vi "Get CD Item Property Value.vi"(8 "error in (no error)":errorcluster, 10 "CD Item Ref in":T1 format="%.0x", 11 "Double Parameter in":refnum<class "Double Array Parameter.lvclass">) -> (0 "error out":errorcluster, 3 "Double Parameter out":refnum<class "Double Array Parameter.lvclass">)   [LabVIEW 2019, in "CD Parameter Manager API.lvlib" / "Double Array Parameter.lvclass"]
uses:
  Double Array Parameter.lvclass
  C:/Repositories/UI-Control-Initializer-API/Source/Parameter Class/Parameter.lvclass
  <vilib>/NI VeriStand/Custom Device API/Custom Device Item Ref.ctl
  Parameter Class/Parameter.lvclass/Parameter.ctl
  Double Array Parameter.lvclass/Double Array Parameter.ctl
  Parameter Class/Member Accessors/Read Control label.vi
  Member Accessors/Read Value.vi
  Member Accessors/Write Value.vi
  <vilib>/NI VeriStand/Custom Device API/Get Item Property (Double Array).vi
  <vilib>/NI VeriStand/Custom Device API/Custom Device API.lvlib
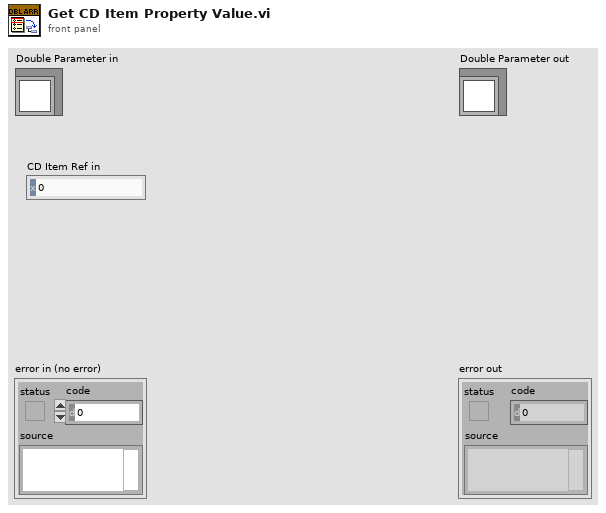
[diagram p1: front panel]
types:
  T1 = typedef "Custom Device API.lvlib/Custom Device Item Ref.ctl" = u64
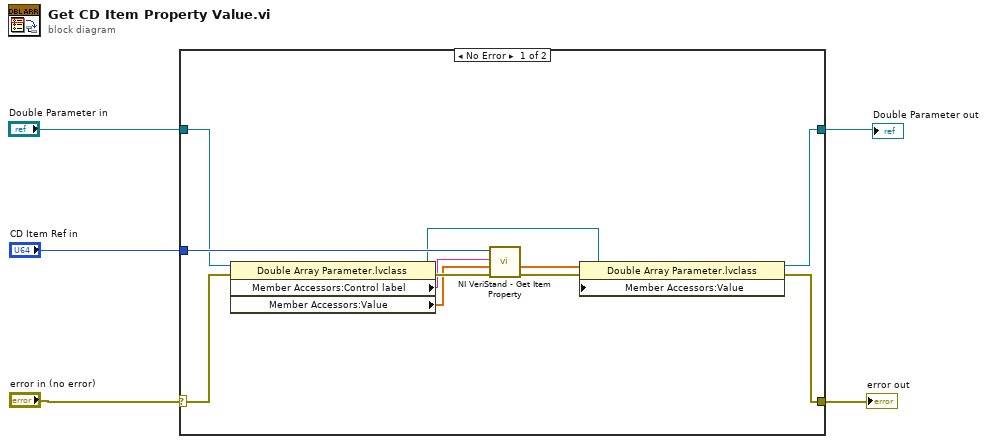
[diagram p0: block diagram]
diagram:
  n1 = case shown="No Error" "error in (no error)" {
    selector: "error in (no error)" -> [w15 w17]
    tunnel: [w11 w17] -> w4
    tunnel: "CD Item Ref in" -> [w16 _]
    tunnel: [w8 w18] -> w5
    tunnel: "Double Parameter in" -> [w7 w18]
    frame No Error {
      n2 = property class="Double Array Parameter.lvclass"(reference=w7, error in=w15) -> (reference out=w9:refnum<class "Double Array Parameter.lvclass">, error out=w14:errorcluster, "Member Accessors:Control label"=w13:string, "Member Accessors:Value"=w6:dbl[])
      n3 = call-poly <vilib>:"NI VeriStand - Get Item Property.vi"("error in (no error)"=w14, "Default Value"=w6, "Property Name"=w13, "Item Ref in"=w16) -> ("error out"=w12:errorcluster, "Value"=w10:dbl[])  [unwired: 4 in, 2 out]
      n4 = property class="Double Array Parameter.lvclass"(reference=w9, error in=w12, "Member Accessors:Value"=w10) -> (reference out=w8:refnum<class "Double Array Parameter.lvclass">, error out=w11:errorcluster)
    }
    frame Error {
    }
  }
  "error out" <- w4
  "Double Parameter out" <- w5
